vi "Read Sub Panel Coin.vi"(8 "error in (no error)":errorcluster, 11 "Monedas USD in":refnum<class "Monedas USD.lvclass">) -> (0 "error out":errorcluster, 2 "Sub Panel Coin":refnum<vi>, 3 "Monedas USD out":refnum<class "Monedas USD.lvclass">)   [LabVIEW 2020, in "Monedas USD.lvlib" / "Monedas USD.lvclass"]
uses:
  Monedas USD.lvclass
  Monedas USD.lvclass/Monedas USD.ctl
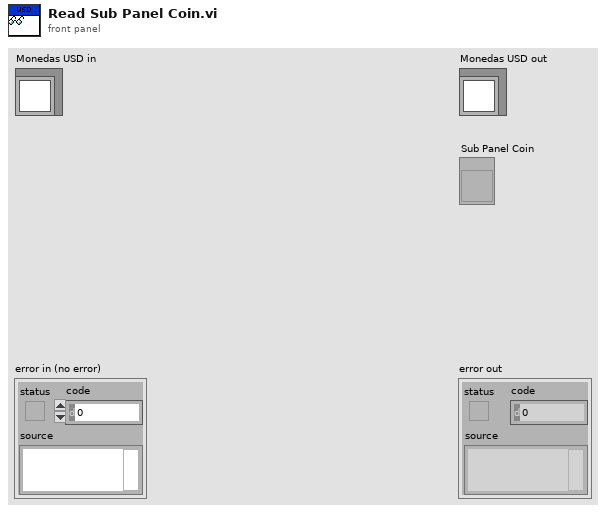
[diagram p1: front panel]
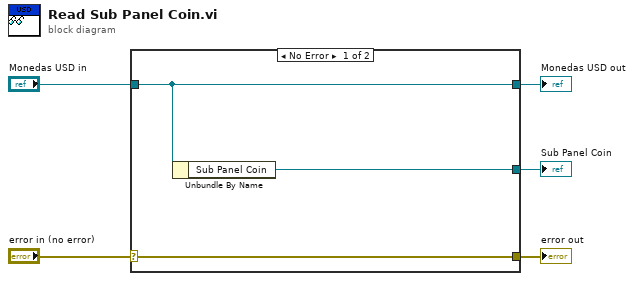
[diagram p0: block diagram]
diagram:
  n1 = case shown="No Error" "error in (no error)" {
    selector: "error in (no error)" -> [w8 w9]
    tunnel: [w8 w9] -> w4
    tunnel: [w7 w10] -> w2
    tunnel: "Monedas USD in" -> [w7 w10]
    tunnel: [w6 _] -> w1
    frame No Error {
      n2 = Unbundle By Name(w7) -> ("Sub Panel Coin"=w6:refnum<vi>)
    }
    frame Error {
    }
  }
  "error out" <- w4
  "Monedas USD out" <- w2
  "Sub Panel Coin" <- w1
